vi "Get AP Sx Ref Curve Val.vi"(0 "asicHandle":i32, 1 "leftX":dbl, 2 "leftY":dbl, 3 "rightX":dbl, 4 "rightY":dbl, 5 "lowerLimit":dbl, 6 "upperLimit":dbl, 7 "error in (no error)":errorcluster caption="错误输入（无错误）", 8 "yScale":dbl) -> (20 "function return":i32, 21 "leftX out":dbl, 22 "leftY out":dbl, 23 "rightX out":dbl, 24 "rightY out":dbl, 25 "lowerLimit out":dbl, 26 "upperLimit out":dbl, 27 "error out":errorcluster caption="错误输出")   [LabVIEW 2018]
doc: "extern int __stdcall GetAPSxRefCurveVal (int asicHandle, OUT double * leftX, OUT double * leftY, OUT double * rightX, OUT double * rightY, OUT double * lowerLimit, OUT double * upperLimit, OUT double yScale);"
uses:
  APSx.dll/APSx.dll
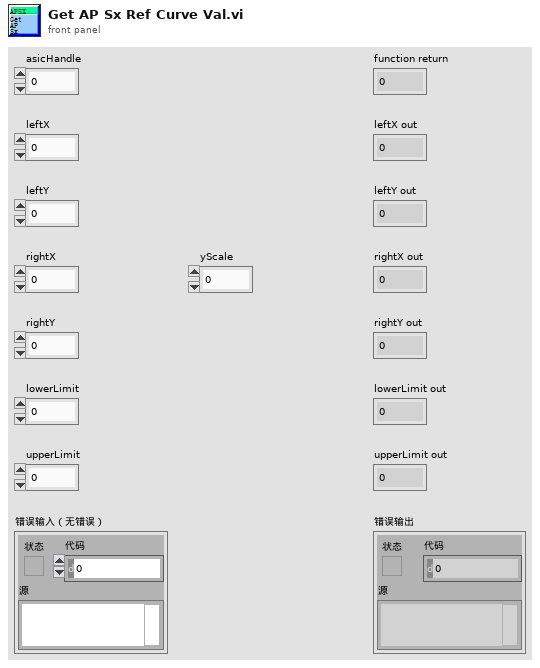
[diagram p1: front panel]
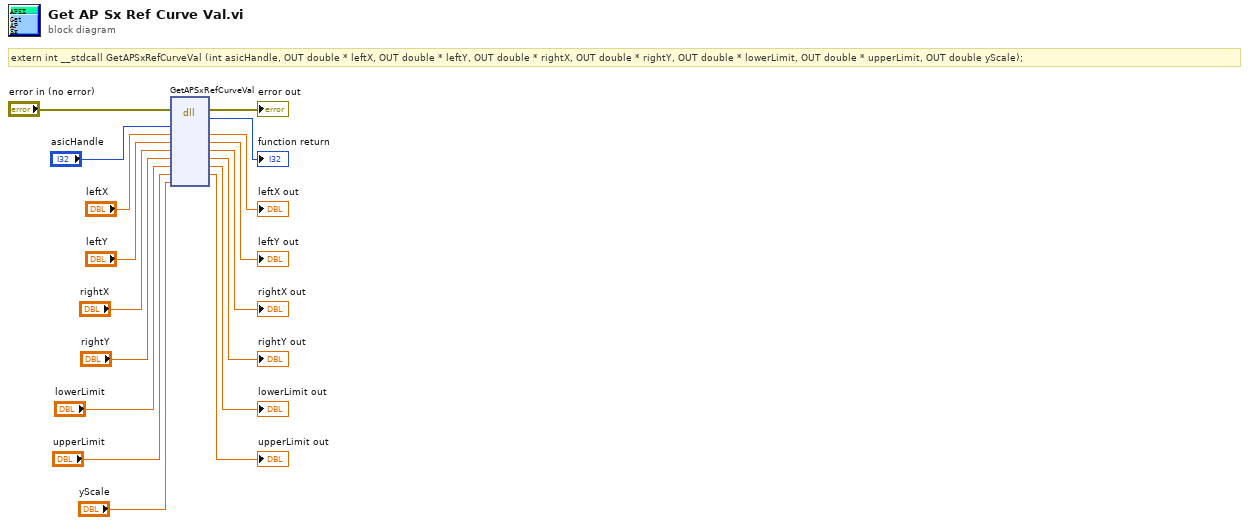
[diagram p0: block diagram]
diagram:
  # "extern int __stdcall GetAPSxRefCurveVal (int asicHandle, OUT double * leftX, OUT double * leftY, OUT double * rightX, OUT double * rightY, OUT double * lowerLimit, OUT double * upperLimit, OUT double yScale);"
  n1 = dll-call lib="PTH2[abs D项目Feng恒隆项目Labview传感器对中台SourcesAPSx.dllAPSx.*" fn="GetAPSxRefCurveVal"(error in="error in (no error)", "asicHandle"="asicHandle", "leftX"="leftX", "leftY"="leftY", "rightX"="rightX", "rightY"="rightY", "lowerLimit"="lowerLimit", "upperLimit"="upperLimit", "yScale"="yScale") -> (error out=→"error out":errorcluster, →"function return":i32, "leftX"=→"leftX out":dbl, "leftY"=→"leftY out":dbl, "rightX"=→"rightX out":dbl, "rightY"=→"rightY out":dbl, "lowerLimit"=→"lowerLimit out":dbl, "upperLimit"=→"upperLimit out":dbl)  [unwired: 4 in, 1 out]
